vi "libssh2_knownhost_readfile - invalid file - returns error.vi"() -> ()   [LabVIEW 2013, in "libssh2_tests.lvlib"]
uses:
  libssh2_tests.lvlib
  libssh2/libssh2_init (Default).vi
  <vilib>/addons/_JKI Toolkits/Caraya/classes/Assert/Assert Error.vi
  <vilib>/addons/_JKI Toolkits/Caraya/classes/Test/Test.lvclass
  libssh2/libssh2.lvlib
  <vilib>/addons/_JKI Toolkits/Caraya/classes/Assert/Assert.lvclass
panel:
  out "error out":errorcluster
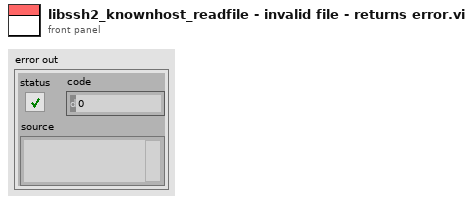
[diagram p1: front panel]
types:
  T1 = typedef "libssh2.lvlib/Session Refnum.ctl" = refnum<k1>
  T2 = typedef "libssh2.lvlib/Known Hosts Refnum.ctl" = refnum<k1>
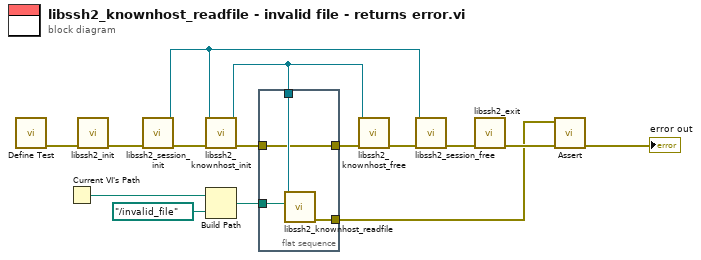
[diagram p0: block diagram]
diagram:
  n1 = call <vilib>:"Define Test.vi"() -> ("error out"=w14:errorcluster)  [unwired: 10 in, 1 out]
  n2 = Current VI's Path() -> (path=w6:path)
  n3 = call-poly "libssh2_init.vi"("error in (no error)"=w14) -> ("error out"=w13:errorcluster)  [unwired: 10 in]
  n4 = call "libssh2_session_init.vi"("error in (no error)"=w13) -> ("error out"=w12:errorcluster, "session"=w9:T1)  [unwired: 9 in]
  n5 = call "libssh2_knownhost_init.vi"("error in (no error)"=w12, "session"=w9) -> ("error out"=w2:errorcluster, "known hosts"=w7:T2)  [unwired: 8 in]
  n6 = Build Path(base path=w6, name or relative path=path "../invalid_file" ("filename")) -> (appended path=w4:path)
  n7 = flat-sequence {
    tunnel: w7 -> [w19]
    tunnel: w4 -> [w18]
    tunnel: [w17] -> w3
    tunnel: w2 -> [w16]
    tunnel: [w16] -> w1
    frame #0 {
      n8 = call "libssh2_knownhost_readfile.vi"("filename"=w18, "known hosts"=w19) -> ("error out"=w17:errorcluster)  [unwired: 8 in, 1 out]
    }
  }
  n9 = call "libssh2_knownhost_free.vi"("error in (no error)"=w1, "known hosts"=w7) -> ("error out"=w8:errorcluster)  [unwired: 9 in]
  n10 = call "libssh2_session_free.vi"("error in (no error)"=w8, "session"=w9) -> ("error out"=w11:errorcluster)  [unwired: 9 in]
  n11 = call "libssh2_exit.vi"("error in (no error)"=w11) -> ("error out"=w10:errorcluster)  [unwired: 10 in]
  n12 = call-poly <vilib>:"Assert.vi"("error in (no error)"=w10, "Error?"=w3) -> ("error out"=→"error out":errorcluster)  [unwired: 8 in, 1 out]
